vi "elapsed_time_calculation.vi"(10 "initial time":u32) -> (2 "elapsed time":dbl)   [LabVIEW 2012]
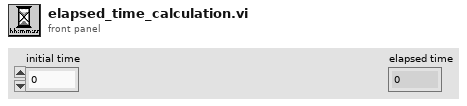
[diagram p1: front panel]
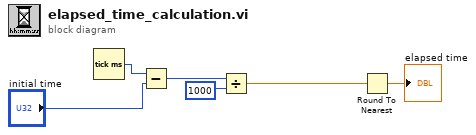
[diagram p0: block diagram]
diagram:
  n1 = Tick Count (ms)() -> (millisecond timer value=w6:u32)
  n2 = Subtract(x=w6, y="initial time") -> (x-y=w5:u32)
  n3 = Divide(x=w5, y=u32 1000) -> (x/y=w3:dbl)
  n4 = Round To Nearest(number=w3) -> (nearest integer value=→"elapsed time":dbl)
